vi "AMI1700_set_meas_mode.vi"(5 "int_samp":i8=15, 7 "mode":enum16{"CONT", "HOLD"}(ring), 8 "error in":errorcluster, 11 "VISA in":refnum<visa-resource-name>) -> (0 "error out":errorcluster, 3 "VISA out":refnum<visa-resource-name>)   [LabVIEW 2019]
panel:
  # "= Sampling interval in minute."
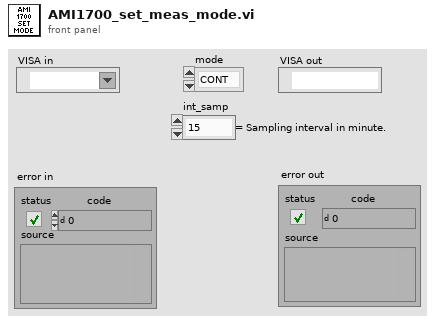
[diagram p1: front panel]
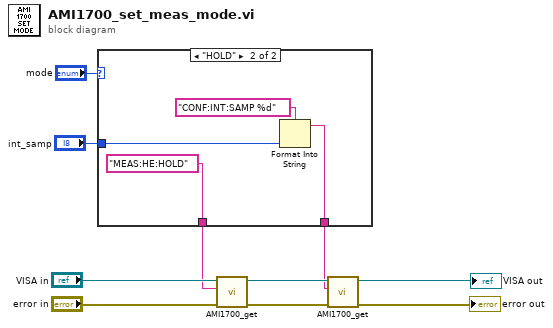
[diagram p0: block diagram]
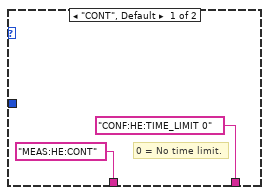
[diagram p2: hidden frame]
diagram:
  n1 = case shown="\"HOLD\"" "mode" {
    tunnel: ["MEAS:HE:CONT" "MEAS:HE:HOLD"] -> w4
    tunnel: ["CONF:HE:TIME_LIMIT 0" ("string in") w13] -> w3
    tunnel: "int_samp" -> [_ w15]
    frame "CONT", Default {
      # "0 = No time limit."
    }
    frame "HOLD" {
      n2 = Format Into String(format string="CONF:INT:SAMP %d" ("string in"), w15) -> (resulting string=w13:string)  [unwired: 2 in, 1 out]
    }
  }
  n3 = call "AMI1700_get.vi"("error in"="error in", "string in"=w4, "VISA in"="VISA in") -> ("error out"=w7:errorcluster, "VISA out"=w8:refnum<visa-resource-name>)  [unwired: 6 in, 1 out]
  n4 = call "AMI1700_get.vi"("error in"=w7, "string in"=w3, "VISA in"=w8) -> ("error out"=→"error out":errorcluster, "VISA out"=→"VISA out":refnum<visa-resource-name>)  [unwired: 6 in, 1 out]
